vi "ReadCSV-R01.vi"(2 "error in (no error)":errorcluster, 3 "CSV path":path=path "C:/LNK213-300/Serial_Log.csv") -> (0 "error out":errorcluster, 1 "Table":string[][](table))   [LabVIEW 2018]
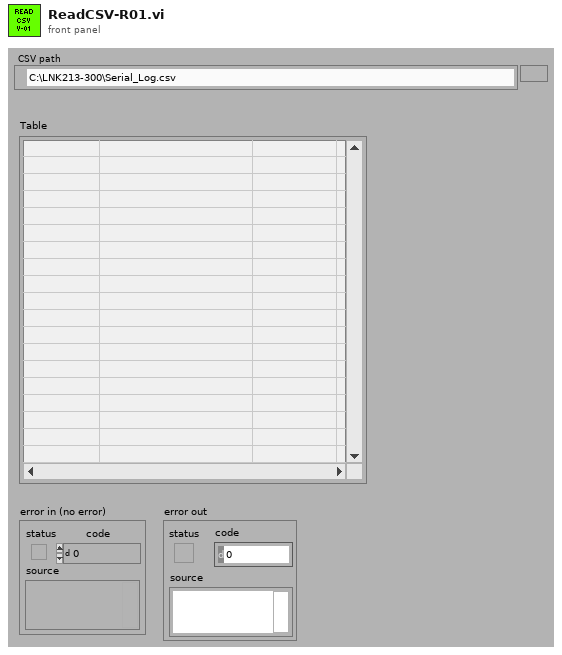
[diagram p1: front panel]
types:
  T1 = enum16{"open", "open or create", "create or replace", "create", "open (read only)"}
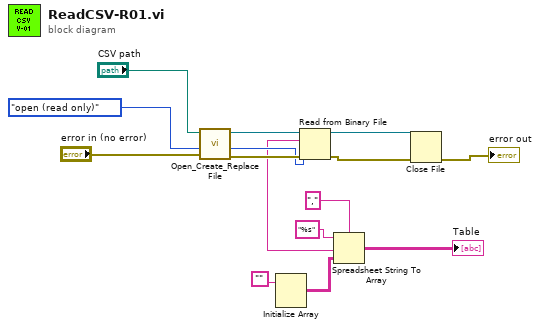
[diagram p0: block diagram]
diagram:
  n1 = call <vilib>:"Open_Create_Replace File.vi"("error in (no error)"="error in (no error)", "function (open:0)"=T1."open (read only)", "file path"="CSV path") -> ("error out"=w12:errorcluster, "file size (bytes)"=w11:i32, "refnum"=w13:refnum<file>)  [unwired: 5 in, 1 out]
  n2 = Initialize Array("") -> (w5:string[][])  [unwired: 2 in]
  n3 = Read from Binary File(8:w12, 10:w11, 11:w13) -> (0:w10:errorcluster, 2:w8:string, 3:w9:refnum<file>)  [unwired: 3 in, 1 out]
  n4 = Spreadsheet String To Array(delimiter (Tab)=",", format string="%s", spreadsheet string=w8, array type (2D Dbl)=w5) -> (array=→"Table":string[][])
  n5 = Close File(refnum=w9, error in=w10) -> (error out=→"error out":errorcluster)  [unwired: 1 out]
